vi "Settings.CreatePerType.vi"(8 "error in (no error)":errorcluster, 10 "Type":T1, 11 "nodeID in":u64) -> (0 "error out":errorcluster, 3 "nodeID out":u64)   [LabVIEW 2019, in "Diagnostics Addon System Explorer.lvlib"]
uses:
  Diagnostics Addon System Explorer.lvlib
  Addon Shared/Types/Type.ctl
  Addon Shared/Diagnostics Addon Shared.lvlib
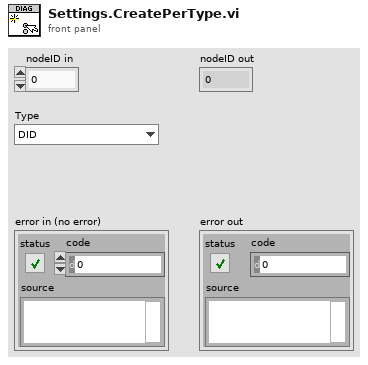
[diagram p1: front panel]
types:
  T1 = typedef "Diagnostics Addon Shared.lvlib/Type.ctl" = enum16{"DID", "CDID", "PID", "CPID", "Read Memory", "Write Memory", "IO Control", "Routine Start", "Routine Request", "Routine Stop", "User Defined", "DTC Control", "Clear DTCs", "Read DTCs", "Start DTCs", "DTC Change Count", "Tester Present", "Unlock ECU", "Reset ECU", "Diag Session Control", "Communication Control", "DPID Control", "Poll Control", "Diag CAN Control"}
  T2 = typedef "Diagnostics Addon Shared.lvlib/Protocol.ctl" = enum16{"GMLAN", "KWP-2000", "UDS", "User-Defined"}
  T3 = typedef "Custom Device API.lvlib/Custom Device Item Ref.ctl" = u64
  T4 = typedef "Diagnostics Addon Shared.lvlib/Settings.Channel.ctl" = cluster{"Name":string, "Description":string, "Channel":T5}
  T5 = typedef "Custom Device API.lvlib/Custom Device Channel.ctl" = cluster{"Type":T6, "Units":string, "Default Value":dbl, "Faultable":bool, "Scalable":bool}
  T6 = typedef "Custom Device API.lvlib/Custom Device Channel Type.ctl" = enum16{"Input", "Output"}
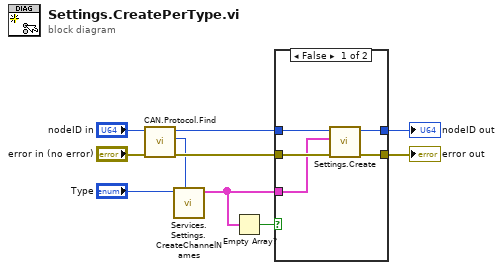
[diagram p0: block diagram]
diagram:
  n1 = call "CAN.Protocol.Find.vi"("error in (no error)"="error in (no error)", "Node Ptr"="nodeID in") -> ("error out"=w6:errorcluster, "Diagnostic Protocol"=w3:T2, "Section Ref out"=w4:T3)  [unwired: 7 in]
  n2 = call "Services.Settings.CreateChannelNames.vi"("Diagnostic Protocol"=w3, "Type"="Type") -> ("Settings Channels"=w10:T4[])  [unwired: 9 in]
  n3 = Empty Array?(array=w10) -> (empty?=w9:bool)
  n4 = case shown="False" w9 {
    tunnel: [w12 w17] -> w1
    tunnel: w4 -> [w14 w17]
    tunnel: [w13 w16] -> w2
    tunnel: w6 -> [w15 w16]
    tunnel: w10 -> [w11 _]
    frame False {
      n5 = call "Settings.Create.vi"("error in (no error)"=w15, "Settings Channels"=w11, "Section Ref in"=w14) -> ("error out"=w13:errorcluster, "nodeID out"=w12:u64)  [unwired: 7 in]
    }
    frame True {
    }
  }
  "error out" <- w2
  "nodeID out" <- w1
